vi "SPC_get_detector_info.vi"(6 "Detector type":i16, 7 "Previous Type":i16 min=0 max=9999 step=1, 8 "Error In":errorcluster, 9 "Last Detector File Name":string, 11 "DLL Path":path) -> (0 "Error Out":errorcluster, 1 "Detector File Name":string, 3 "DLL Path":path, 4 "Detector Type":i16 min=0 max=9999 step=1, 5 "Previous Type":i16)   [LabVIEW 2023]
doc: "The procedure is used to look for specific detector type on the detectors list for SPC-930 module.\n\nFor further information please take a look into the 'spcmdll.pdf\".\n\nOctober 2018\nFrank Quadt & Stefan Smietana\ninfo@becker-hickl.com"
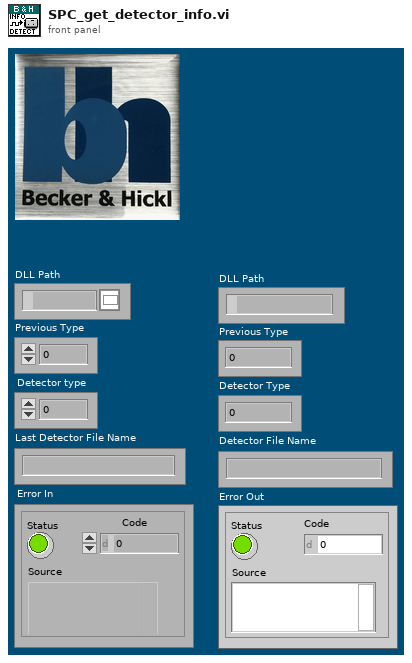
[diagram p1: front panel]
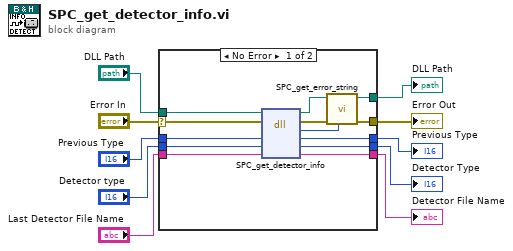
[diagram p0: block diagram]
diagram:
  n1 = case shown="No Error" "Error In" {
    selector: "Error In" -> [w21 w28]
    tunnel: "DLL Path" -> [w23 w27]
    tunnel: [w17 w27] -> w9
    tunnel: [w22 w28] -> w8
    tunnel: [w16 w26] -> w6
    tunnel: [w15 w24] -> w5
    tunnel: "Previous Type" -> [w14 w25]
    tunnel: "Last Detector File Name" -> [w13 w26]
    tunnel: "Detector type" -> [w12 w24]
    tunnel: [w11 w25] -> w1
    frame No Error {
      n2 = dll-call lib="D:/spcm/lib/lab_view/lv10.0/spcm32.dll" fn="SPC_get_detector_info"(path in=w23, error in=w21, "previous_type"=w14, "det_type"=w12, "fname"=w13) -> (path out=w18:path, error out=w20:errorcluster, "return type"=w19:i16, "previous_type"=w11:i16, "det_type"=w15:i16, "fname"=w16:string)  [unwired: 1 in]
      n3 = call "SPC_get_error_string.vi"("ErrorID"=w19, "Error In"=w20, "DLL Path"=w18) -> ("Error Out"=w22:errorcluster, "DLL Path"=w17:path)  [unwired: 6 in, 1 out]
    }
    frame Error {
    }
  }
  "DLL Path" <- w9
  "Error Out" <- w8
  "Detector File Name" <- w6
  "Detector Type" <- w5
  "Previous Type" <- w1
